vi "Init Dynamixel Serial.vi"(11 "VISA Refnum in":refnum<visa-resource-name>) -> (0 "error out":errorcluster, 3 "VISA Refnum out":refnum<visa-resource-name>)   [LabVIEW 2013]
doc: "This VI should intialize the Dynamixels. That might involve discovering which IDs they have and resetting them to the correct IDs. That might also involve discovering what comm rates they're on and resetting those.\n\nEric Schneider, April 2014"
uses:
  <instrlib>/Dynamixel Motor/Dynamixel Motor.lvlib
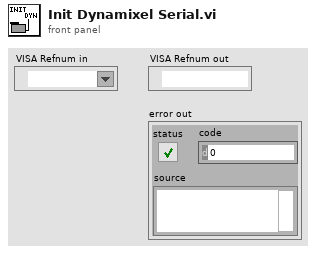
[diagram p1: front panel]
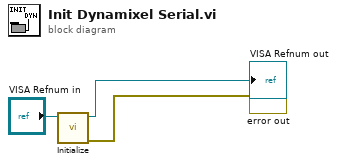
[diagram p0: block diagram]
diagram:
  n1 = call <instrlib>:"Initialize.vi"("VISA resource name"="VISA Refnum in") -> ("error out"=→"error out":errorcluster, "VISA resource name out"=→"VISA Refnum out":refnum<visa-resource-name>)  [unwired: 9 in]
